vi "ArduinoToInt (SubVI).vi"(10 "Byte Array of Ardunio String":i32[](array[numeric]), 11 "Length of Ardunio Output":i32) -> (1 "String":string, 2 "Numeric":i32, 3 "Array":i32[](array[numeric]))   [LabVIEW 2017]
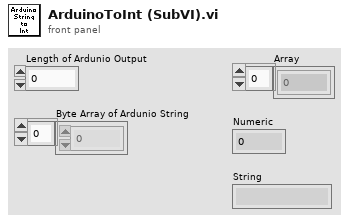
[diagram p1: front panel]
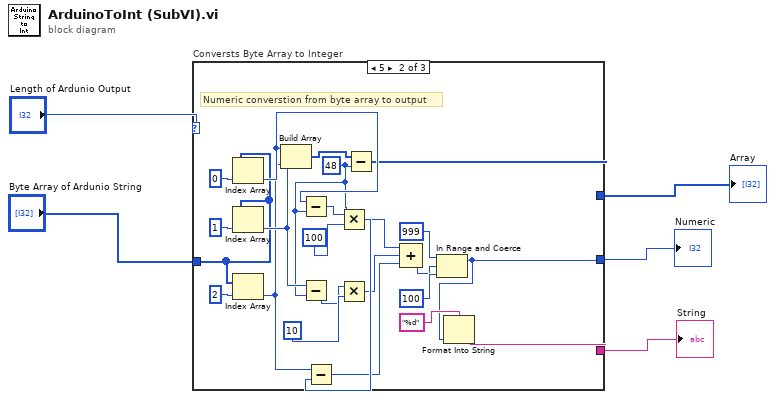
[diagram p0: block diagram]
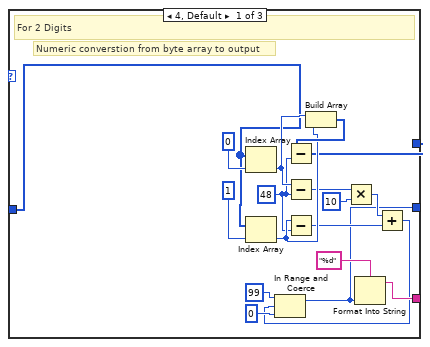
[diagram p2: hidden frame]
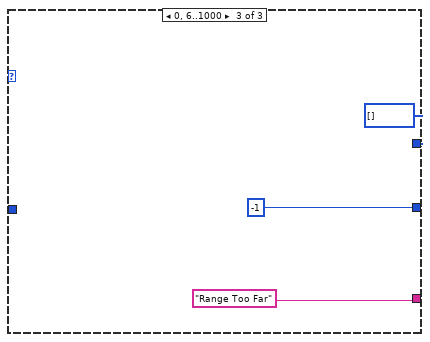
[diagram p3: hidden frame]
diagram:
  n1 = case "Conversts Byte Array to Integer" shown="5" "Length of Ardunio Output" {
    tunnel: [w8 w26 -1] -> w3
    tunnel: [w15 w35 "Range Too Far"] -> w2
    tunnel: "Byte Array of Ardunio String" -> [w7 w25 _]
    tunnel: [w6 w24 i32[] []] -> w5
    frame 4, Default {
      w18 = 48
      # "Numeric converstion from byte array to output"
      # "For 2 Digits"
      n2 = Index Array(array=w7, index=0) -> (element=w20:i32)
      n3 = Index Array(array=w7, index=1) -> (element=w19:i32)
      n4 = Subtract(x=w20, y=w18) -> (x-y=w13:i32)
      n5 = Subtract(x=w19, y=w18) -> (x-y=w12:i32)
      n6 = Build Array(w20, w19) -> (w21:i32[])
      n7 = Subtract(x=w21, y=w18) -> (x-y=w6:i32[])
      n8 = Multiply(x=w13, y=10) -> (x*y=w16:i32)
      n9 = Add(x=w16, y=w12) -> (x+y=w9:i32)
      n10 = In Range and Coerce(upper limit=99, x=w9, lower limit=0) -> (coerced(x)=w8:i32)  [unwired: 1 out]
      n11 = Format Into String(format string="%d", w8) -> (resulting string=w15:string)  [unwired: 2 in, 1 out]
    }
    frame 5 {
      w37 = 48
      # "Numeric converstion from byte array to output"
      n12 = Index Array(array=w25, index=0) -> (element=w42:i32)
      n13 = Index Array(array=w25, index=1) -> (element=w40:i32)
      n14 = Index Array(array=w25, index=2) -> (element=w38:i32)
      n15 = Build Array(w42, w40, w38) -> (w43:i32[])
      n16 = Subtract(x=w42, y=w37) -> (x-y=w31:i32)
      n17 = Subtract(x=w40, y=w37) -> (x-y=w30:i32)
      n18 = Subtract(x=w38, y=w37) -> (x-y=w32:i32)
      n19 = Multiply(x=w31, y=100) -> (x*y=w34:i32)
      n20 = Multiply(x=w30, y=10) -> (x*y=w33:i32)
      n21 = Subtract(x=w43, y=w37) -> (x-y=w24:i32[])
      n22 = Compound Arithmetic op=ADD(w34, w33, w32) -> (w27:i32)
      n23 = In Range and Coerce(upper limit=999, x=w27, lower limit=100) -> (coerced(x)=w26:i32)  [unwired: 1 out]
      n24 = Format Into String(format string="%d", w26) -> (resulting string=w35:string)  [unwired: 2 in, 1 out]
    }
    frame 0, 6..1000 {
    }
  }
  "Array" <- w5
  "Numeric" <- w3
  "String" <- w2
